vi "Get MultiColumn Listbox click row index.vi"(8 "error in (no error)":errorcluster, 10 "Coords":T2, 11 "CtlRef":refnum<vi>) -> (0 "error out":errorcluster, 1 "subarray":string[](array[string]), 2 "Cell Position":T1, 3 "CtlRef Out":refnum<vi>, 5 "Row":i32)   [LabVIEW 2021]
uses:
  <vilib>/Utility/miscctls.llb/LVPoint32TypeDef.ctl
  <vilib>/Utility/miscctls.llb/LVRowAndColumnTypeDef.ctl
  <vilib>/Utility/miscctls.llb/LVPositionTypeDef.ctl
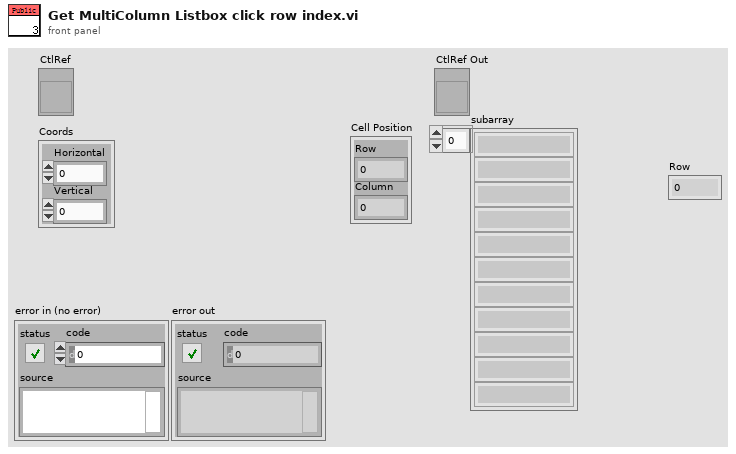
[diagram p1: front panel]
types:
  T1 = typedef "LVRowAndColumnTypeDef.ctl" = cluster{"Row":i32, "Column":i32}
  T2 = typedef "LVPoint32TypeDef.ctl" = cluster{"Horizontal":i32, "Vertical":i32}
  T3 = typedef "LVPositionTypeDef.ctl" = cluster{"Left":i32, "Top":i32}
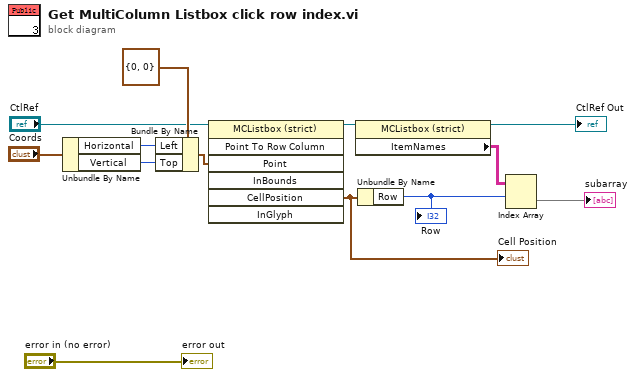
[diagram p0: block diagram]
diagram:
  n1 = Unbundle By Name("Coords") -> ("Horizontal"=w8:i32, "Vertical"=w9:i32)
  n2 = Bundle By Name(cluster=T3 {"Left"=0, "Top"=0} ("Point"), "Left"=w8, "Top"=w9) -> (w1:T3)
  n3 = invoke class="MCListbox (strict)" method="Point To Row Column"(reference="CtlRef", "Point"=w1) -> (reference out=w10:refnum<vi>, "CellPosition"=w12:T1)  [unwired: 5 in, 5 out]
  "Cell Position" <- w12
  n4 = property class="MCListbox (strict)"(reference=w10) -> (reference out=→"CtlRef Out":refnum<vi>, "ItemNames"=w11:string[][])  [unwired: 1 in, 1 out]
  n5 = Unbundle By Name(w12) -> ("Row"=w13:i32)
  "Row" <- w13
  n6 = Index Array(array=w11, index (row)=w13) -> (element=→"subarray":string[])  [unwired: 1 in]
  "error out" <- "error in (no error)"
